vi "SRV_Update Front Panel Window Title.vi"(7 "Window Title Override String":string, 8 "error in (no error)":errorcluster, 11 "VI ref":refnum<vi>) -> (0 "error out":errorcluster, 3 "VI ref out":refnum<vi>)   [LabVIEW 2009]
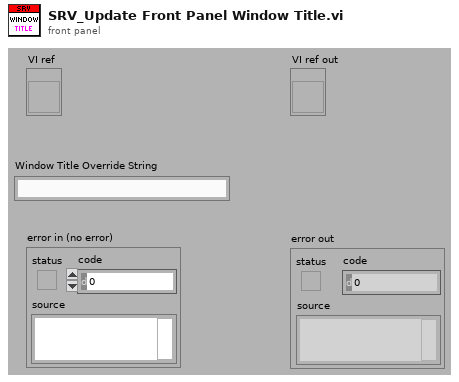
[diagram p1: front panel]
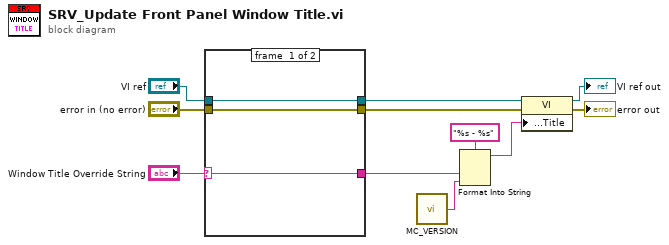
[diagram p0: block diagram]
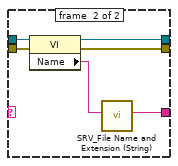
[diagram p2: hidden frame]
diagram:
  n1 = case shown="\"\"" "Window Title Override String" {
    selector: "Window Title Override String" -> [w12 _]
    tunnel: "error in (no error)" -> [w13 w20]
    tunnel: "VI ref" -> [w14 w19]
    tunnel: [w12 w17] -> w8
    tunnel: [w14 w16] -> w6
    tunnel: [w13 w15] -> w2
    frame #0 {
    }
    frame #1 {
      n2 = property class="VI"(reference=w19, error in=w20) -> (reference out=w16:refnum<vi>, error out=w15:errorcluster, "Name"=w18:string)
      n3 = call "SRV_File Name and Extension (String).vi"("File or Directory String"=w18) -> ("Name"=w17:string)  [unwired: 9 in, 1 out]
    }
  }
  n4 = call "MC_VERSION.vi"() -> ("MC Version"=w7:string)
  n5 = Format Into String(format string="%s - %s", w8, w7) -> (resulting string=w3:string)  [unwired: 2 in, 1 out]
  n6 = property class="VI"(reference=w6, error in=w2, "Front Panel.Title"=w3) -> (reference out=→"VI ref out":refnum<vi>, error out=→"error out":errorcluster)
